vi "电源管理UI.vi"() -> ()   [LabVIEW 2016, in "PLC.lvlib"]
uses:
  PLC.lvlib
  <vilib>/Utility/miscctls.llb/LVPointTypeDef.ctl
panel:
  in  "看门狗启用":bool
  out "R123":i16 caption="看门狗设置"
  out "R56":i16 caption="看门狗计时器"
  in  "自动运行启动参数":T1
  # "S"
  # "S"
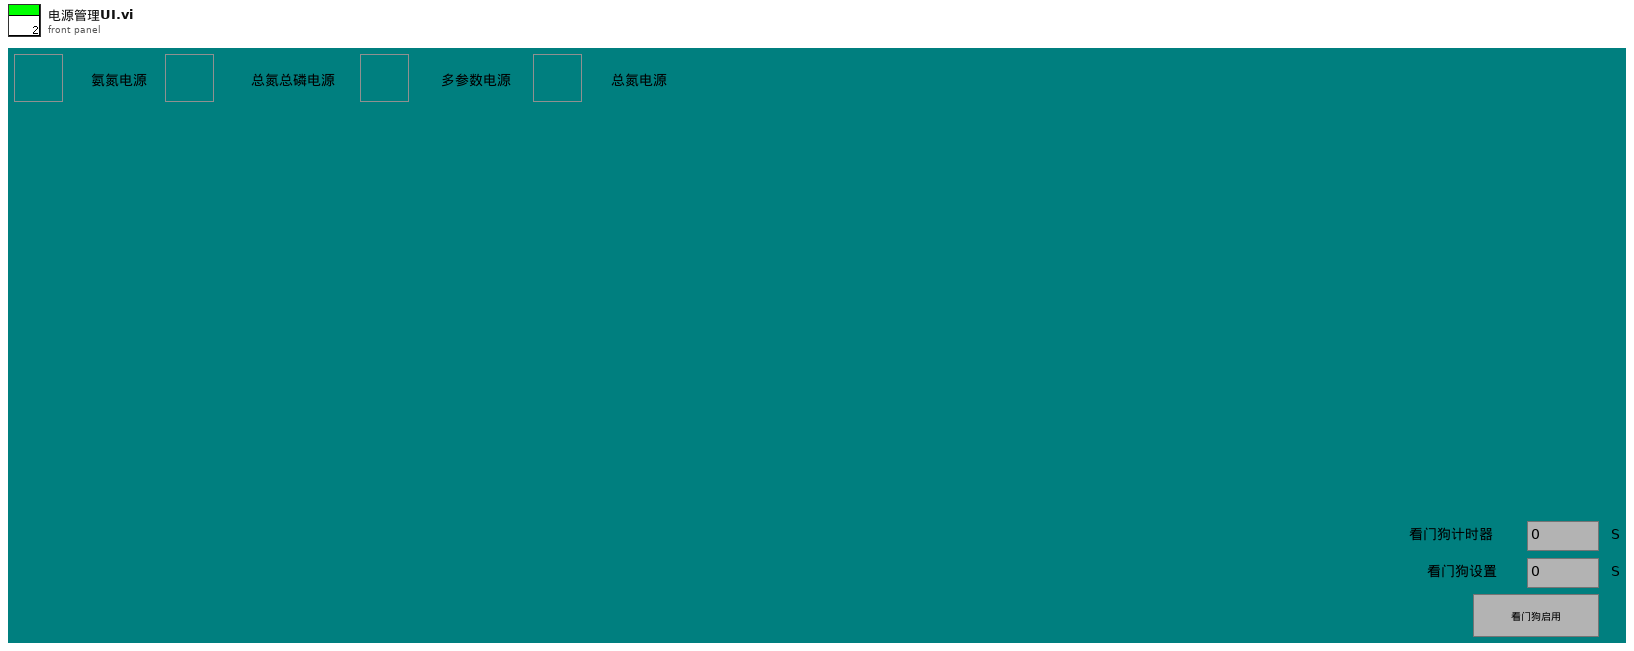
[diagram p1: front panel]
types:
  T1 = cluster{"氨氮":bool, "总磷总氮":bool, "CODmn":bool, "CODCr":bool, "多参数":bool, "总氮电源":bool}
  T2 = typedef "LVPointTypeDef.ctl" = cluster{"Horizontal":i16, "Vertical":i16}
  T3 = cluster{"R100":i16, "R101":i16, "R102":i16, "R103":i16, "R104":i16, "R105":i16, "R106":i16, "R107":i16, "R108":i16, "R109":i16, "R110":i16, "R111":i16, "R112":i16, "R113":i16, "R114":i16, "R115":i16, "R116":i16, "R117":i16, "R118":i16, "R119":i16, "R120":i16, "R121":i16, "R122":i16, "R123":i16, "R124":i16}
  T4 = cluster{"R0":i16, "R1":i16, "R2":i16, "R3":i16, "R4":i16, "R5":i16, "R6":i16, "R7":i16, "R8":i16, "R9":i16, "R10":i16, "R11":i16, "R12":i16, "R13":i16, "R14":i16, "R15":i16, "R16":i16, "R17":i16, "R18":i16, "R19":i16, "R20":i16, "R21":i16, "R22":i16, "R23":i16, "R24":i16, "R25":i16, "R26":i16, "R27":i16, "R28":i16, "R29":i16, "R30":i16, "R31":i16, "R32":i16, "R33":i16, "R34":i16, "R35":i16, "R36":i16, "R37":i16, "R38":i16, "R39":i16, "R40":i16, "R41":i16, "R42":i16, "R43":i16, "R44":i16, "R45":i16, "R46":i16, "R47":i16, "R48":i16, "R49":i16, "R50":i16, "R51":i16, "R52":i16, "R53":i16, "R54":i16, "R55":i16, "R56":i16}
  T5 = cluster{"命令":string, "数据":cluster{"starting address":u16, "holding register values":u16[]}}
  T6 = cluster{"命令":string, "data":cluster{"starting address":u16, "coil values":bool[]}}
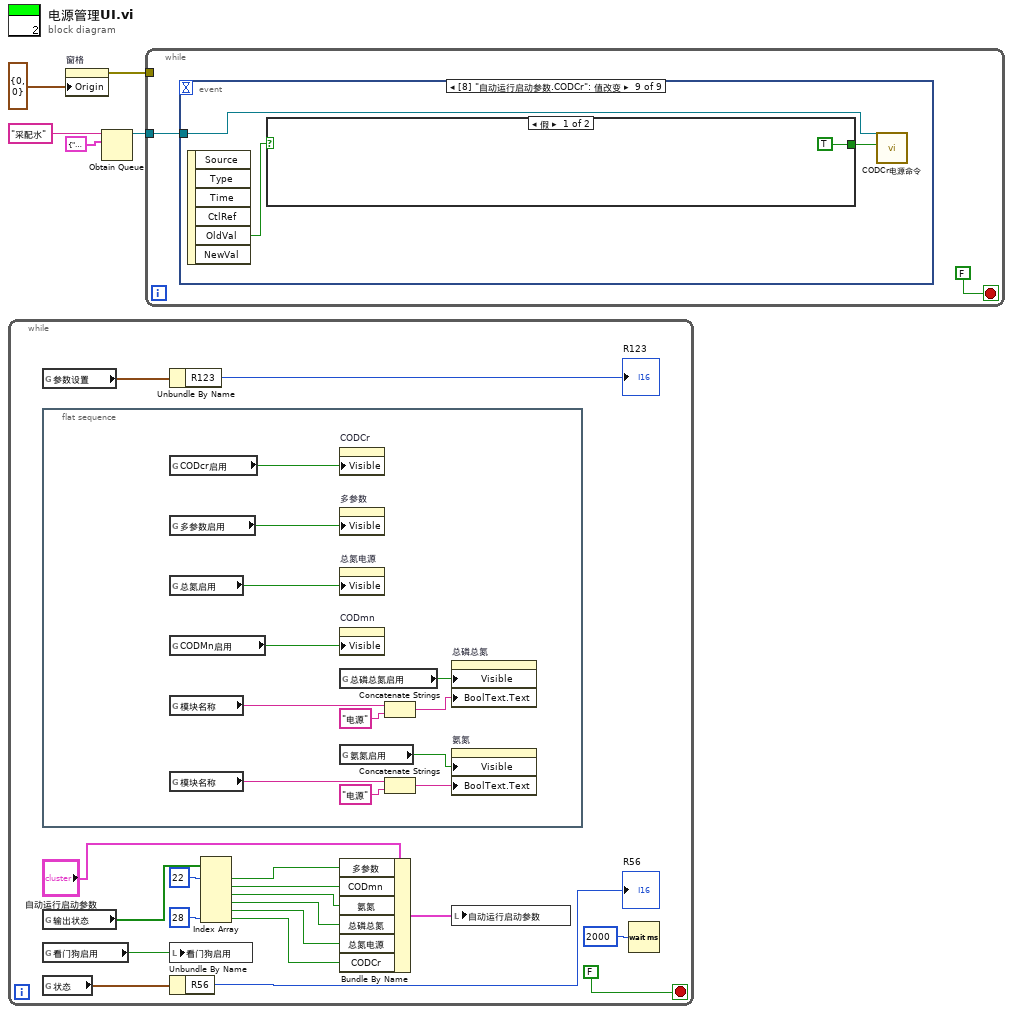
[diagram p0: block diagram]
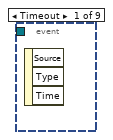
[diagram p2: hidden frame]
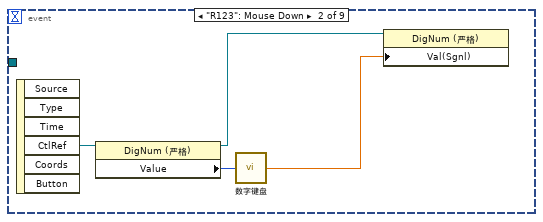
[diagram p3: hidden frame]
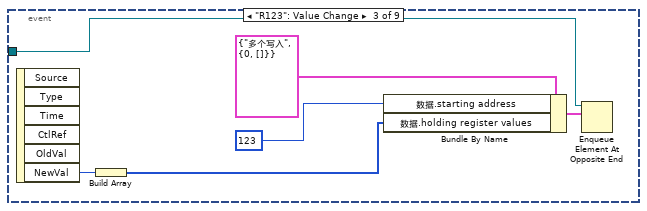
[diagram p4: hidden frame]
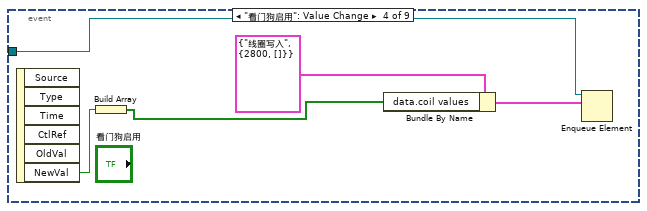
[diagram p5: hidden frame]
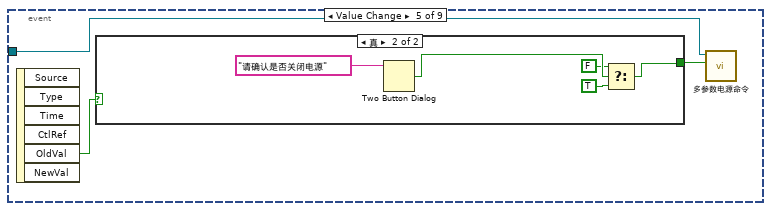
[diagram p6: hidden frame]
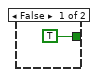
[diagram p7: hidden frame]
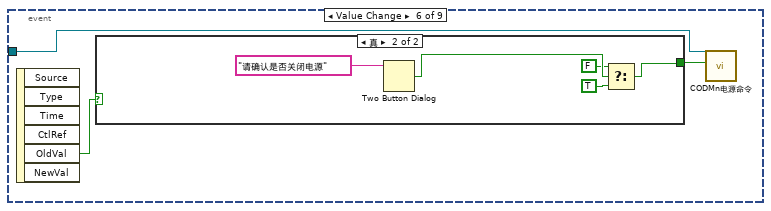
[diagram p8: hidden frame]
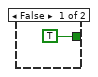
[diagram p9: hidden frame]
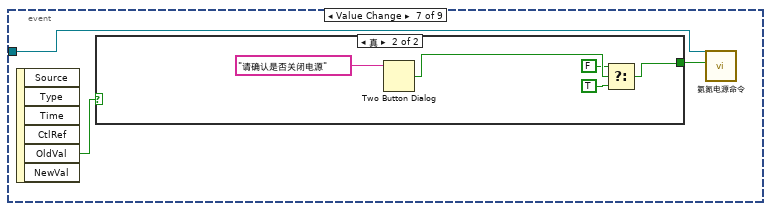
[diagram p10: hidden frame]
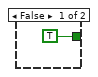
[diagram p11: hidden frame]
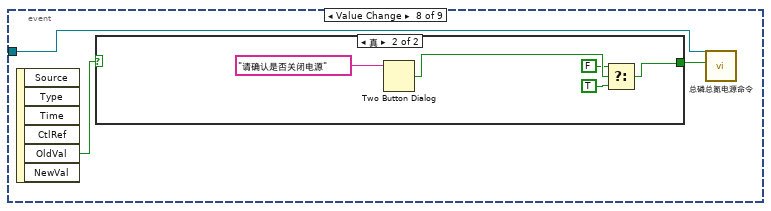
[diagram p12: hidden frame]
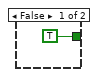
[diagram p13: hidden frame]
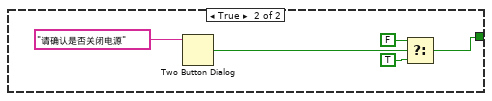
[diagram p14: hidden frame]
diagram:
  n1 = while {
    stop <- FALSE stop-if-true
    n2 = global read "采配水全局变量.vi" "参数设置"() -> (w12:T3)
    n3 = flat-sequence {
      frame #0 {
        n4 = global read "系统设置全局变量.vi" "CODcr启用"() -> (w28:bool)
        n5 = global read "系统设置全局变量.vi" "多参数启用"() -> (w34:bool)
        n6 = global read "系统设置全局变量.vi" "总氮启用"() -> (w29:bool)
        n7 = global read "系统设置全局变量.vi" "CODMn启用"() -> (w32:bool)
        n8 = global read "VAR总磷总氮全局变量.vi" "模块名称"() -> (w27:string)
        n9 = global read "VAR总磷总氮全局变量.vi" "模块名称"() -> (w25:string)
        n10 = property on="CODCr" class="Bool (严格)"("Visible"=w28) -> ()  [unwired: 2 in, 2 out]
        n11 = property on="多参数" class="Bool (严格)"("Visible"=w34) -> ()  [unwired: 2 in, 2 out]
        n12 = property on="总氮电源" class="Bool (严格)"("Visible"=w29) -> ()  [unwired: 2 in, 2 out]
        n13 = property on="CODmn" class="Bool (严格)"("Visible"=w32) -> ()  [unwired: 2 in, 2 out]
        n14 = global read "系统设置全局变量.vi" "总磷总氮启用"() -> (w33:bool)
        n15 = global read "系统设置全局变量.vi" "氨氮启用"() -> (w35:bool)
        n16 = Concatenate Strings(w27, "电源" ("字符串")) -> (w30:string)
        n17 = Concatenate Strings(w25, "电源" ("字符串")) -> (w24:string)
        n18 = property on="总磷总氮" class="Bool (严格)"("Visible"=w33, "BoolText.Text"=w30) -> ()  [unwired: 2 in, 2 out]
        n19 = property on="氨氮" class="Bool (严格)"("Visible"=w35, "BoolText.Text"=w24) -> ()  [unwired: 2 in, 2 out]
      }
    }
    n20 = global read "采配水全局变量.vi" "输出状态"() -> (w21:bool[])
    n21 = global read "采配水全局变量.vi" "看门狗启用"() -> (w13:bool)
    n22 = global read "采配水全局变量.vi" "状态"() -> (w10:T4)
    n23 = Unbundle By Name(w12) -> ("R123"=→"R123":i16)
    n24 = local write "看门狗启用"(w13) -> ()
    n25 = Unbundle By Name(w10) -> ("R56"=→"R56":i16)
    n26 = Index Array(array=w21, index #1=22 ("索引"), index #6=28 ("索引")) -> (element #1=w18:bool, element #2=w17:bool, element #3=w16:bool, element #4=w15:bool, element #5=w6:bool, element #6=w7:bool)  [unwired: 4 in]
    n27 = Bundle By Name(cluster="自动运行启动参数", "多参数"=w18, "CODmn"=w17, "氨氮"=w16, "总磷总氮"=w15, "总氮电源"=w6, "CODCr"=w7) -> (w14:T1)
    n28 = local write "自动运行启动参数"(w14) -> ()
    n29 = Wait (ms)(milliseconds to wait=u32 2000 ("等待时间（毫秒）")) -> ()  [unwired: 1 out]
  }
  n30 = property on="窗格" class="Pane"("Origin"=T2 {"Horizontal"=0, "Vertical"=0} ("原点")) -> (error out=w2:errorcluster)  [unwired: 2 in, 1 out]
  n31 = Obtain Queue(name (unnamed)="采配水" ("名称（未命名）"), element data type=cluster{"命令":string, "数据":variant} {"命令"="", "数据"=variant}) -> (queue out=w1:refnum<queue>)  [unwired: 3 in, 2 out]
  n32 = while {
    tunnel: w1 -> [w36]
    tunnel: w2 -> [_]
    stop <- FALSE stop-if-true
    n33 = event shown="[8] \"自动运行启动参数.CODCr\": 值改变" {
      selector: _ -> [_ _ _ _ _ _ _ _ _]
      dyn-events: _ -> [_ _ _ _ _ _ _ _ _]
      timeout: _ -> [_ _ _ _ _ _ _ _ _]
      tunnel: w36 -> [_ _ w42 w48 w55 w64 w73 w82 w91]
      event Timeout {
        n34 = event-data() -> ()  [unwired: 1 in, 3 out]
      }
      event "R123": Mouse Down {
        n35 = event-data() -> ("CtlRef"=w41:refnum<vi>)  [unwired: 1 in, 5 out]
        n36 = property class="DigNum (严格)"(reference=w41) -> (reference out=w40:refnum<vi>, "Value"=w39:i16)  [unwired: 1 in, 1 out]
        n37 = call "数字键盘.vi"("OldNumber"=w39) -> ("NewNumber"=w38:sgl)
        n38 = property class="DigNum (严格)"(reference=w40, "Val(Sgnl)"=w38) -> ()  [unwired: 1 in, 2 out]
      }
      event "R123": Value Change {
        n39 = event-data() -> ("NewVal"=w44:i16)  [unwired: 1 in, 5 out]
        n40 = Build Array(w44) -> (w43:i16[])
        n41 = Bundle By Name(cluster=T5 {"命令"="多个写入", "数据"={"starting address"=0, "holding register values"=[]}} ("元素"), "数据.starting address"=u16 123, "数据.holding register values"=w43) -> (w45:T5)
        n42 = Enqueue Element At Opposite End(queue=w42, element=w45) -> ()  [unwired: 2 in, 3 out]
      }
      event "看门狗启用": Value Change {
        n43 = event-data() -> ("NewVal"=w50:bool)  [unwired: 1 in, 5 out]
        n44 = Build Array(w50) -> (w49:bool[])
        n45 = Bundle By Name(cluster=T6 {"命令"="线圈写入", "data"={"starting address"=2800, "coil values"=[]}} ("元素"), "data.coil values"=w49) -> (w51:T6)
        n46 = Enqueue Element(queue=w48, element=w51) -> ()  [unwired: 2 in, 3 out]
      }
      event "自动运行启动参数.多参数": Value Change {
        n47 = event-data() -> ("OldVal"=w54:bool)  [unwired: 1 in, 5 out]
        n48 = case shown="真" w54 {
          tunnel: [TRUE ("T button?") w57] -> w53
          frame False {
          }
          frame True {
            n49 = Two Button Dialog(message="请确认是否关闭电源" ("消息")) -> (T button?=w60:bool)  [unwired: 2 in]
            n50 = Select(t=FALSE, s=w60, f=TRUE ("T button?")) -> (s? t:f=w57:bool)
          }
        }
        n51 = call "多参数电源命令.vi"("通电/断电"=w53, "队列"=w55) -> ()  [unwired: 9 in, 1 out]
      }
      event "自动运行启动参数.CODmn": Value Change {
        n52 = event-data() -> ("OldVal"=w63:bool)  [unwired: 1 in, 5 out]
        n53 = case shown="真" w63 {
          tunnel: [TRUE ("T button?") w66] -> w62
          frame False {
          }
          frame True {
            n54 = Two Button Dialog(message="请确认是否关闭电源" ("消息")) -> (T button?=w69:bool)  [unwired: 2 in]
            n55 = Select(t=FALSE, s=w69, f=TRUE ("T button?")) -> (s? t:f=w66:bool)
          }
        }
        n56 = call "CODMn电源命令.vi"("通电/断电"=w62, "队列"=w64) -> ()  [unwired: 9 in, 1 out]
      }
      event "自动运行启动参数.氨氮": Value Change {
        n57 = event-data() -> ("OldVal"=w72:bool)  [unwired: 1 in, 5 out]
        n58 = case shown="真" w72 {
          tunnel: [TRUE ("T button?") w75] -> w71
          frame False {
          }
          frame True {
            n59 = Two Button Dialog(message="请确认是否关闭电源" ("消息")) -> (T button?=w78:bool)  [unwired: 2 in]
            n60 = Select(t=FALSE, s=w78, f=TRUE ("T button?")) -> (s? t:f=w75:bool)
          }
        }
        n61 = call "氨氮电源命令.vi"("通电/断电"=w71, "队列"=w73) -> ()  [unwired: 9 in, 1 out]
      }
      event "自动运行启动参数.总磷总氮": Value Change {
        n62 = event-data() -> ("OldVal"=w81:bool)  [unwired: 1 in, 5 out]
        n63 = case shown="真" w81 {
          tunnel: [TRUE ("T button?") w84] -> w80
          frame False {
          }
          frame True {
            n64 = Two Button Dialog(message="请确认是否关闭电源" ("消息")) -> (T button?=w87:bool)  [unwired: 2 in]
            n65 = Select(t=FALSE, s=w87, f=TRUE ("T button?")) -> (s? t:f=w84:bool)
          }
        }
        n66 = call "总磷总氮电源命令.vi"("通电/断电"=w80, "队列"=w82) -> ()  [unwired: 9 in, 1 out]
      }
      event "自动运行启动参数.CODCr": Value Change {
        n67 = event-data() -> ("OldVal"=w90:bool)  [unwired: 1 in, 5 out]
        n68 = case shown="假" w90 {
          tunnel: [TRUE ("T button?") w93] -> w89
          frame False {
          }
          frame True {
            n69 = Two Button Dialog(message="请确认是否关闭电源" ("消息")) -> (T button?=w96:bool)  [unwired: 2 in]
            n70 = Select(t=FALSE, s=w96, f=TRUE ("T button?")) -> (s? t:f=w93:bool)
          }
        }
        n71 = call "CODCr电源命令.vi"("通电/断电"=w89, "队列"=w91) -> ()  [unwired: 9 in, 1 out]
      }
    }
  }
